vi "overlap_calculator.vi"(0 "T1":dbl min=0.0, 2 "T2":dbl min=0.0, 3 "D":dbl min=0.0) -> (6 "overlap":dbl, 10 "delay":dbl)   [LabVIEW 2015]
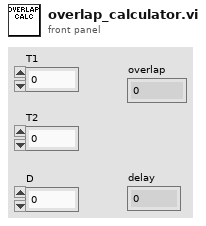
[diagram p1: front panel]
types:
  T1 = enum16{"D<=T1-T2 ^ D<T1", "D<T1 ^ D>T1-T2", "D>=T1"}
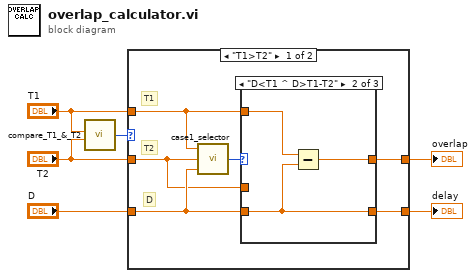
[diagram p0: block diagram]
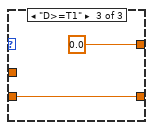
[diagram p3: hidden frame]
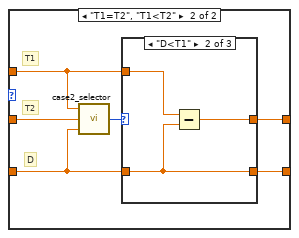
[diagram p4: hidden frame]
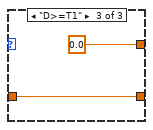
[diagram p6: hidden frame]
diagram:
  n1 = call "compare_T1_&_T2.vi"("T1"="T1", "T2"="T2") -> ("Result"=w2:enum16{"T1>T2", "T1=T2", "T1<T2"})  [unwired: 6 in]
  n2 = case shown="\"T1>T2\"" w2 {
    tunnel: "T1" -> [w10 w23]
    tunnel: "T2" -> [w8 w25]
    tunnel: "D" -> [w9 w21]
    tunnel: [w11 w22] -> w6
    tunnel: [w7 w20] -> w1
    frame "T1>T2" {
      # "D"
      # "T2"
      # "T1"
      n3 = call "case1_selector.vi"("T1"=w10, "T2"=w8, "Delay"=w9) -> ("overlap select"=w12:T1)  [unwired: 4 in]
      n4 = case shown="\"D<T1 ^ D>T1-T2\"" w12 {
        tunnel: w10 -> [_ w17 _]
        tunnel: [w14 w16 0.0] -> w11
        tunnel: w9 -> [w13 w15 w18]
        tunnel: w8 -> [w14 _ _]
        tunnel: [w13 w15 w18] -> w7
        frame "D<=T1-T2 ^ D<T1" {
        }
        frame "D<T1 ^ D>T1-T2" {
          n5 = Subtract(x=w17, y=w15) -> (x-y=w16:dbl)
        }
        frame "D>=T1" {
        }
      }
    }
    frame "T1=T2", "T1<T2" {
      # "D"
      # "T2"
      # "T1"
      n6 = call "case2_selector.vi"("T1"=w23, "T2"=w25, "Delay"=w21) -> ("Case 2 selector"=w24:enum16{"D=0", "D<T1", "D>=T1"})  [unwired: 4 in]
      n7 = case shown="\"D<T1\"" w24 {
        tunnel: w23 -> [w27 w29 _]
        tunnel: [w27 w30 0.0] -> w22
        tunnel: w21 -> [w26 w28 w31]
        tunnel: [w26 w28 w31] -> w20
        frame "D=0" {
        }
        frame "D<T1" {
          n8 = Subtract(x=w29, y=w28) -> (x-y=w30:dbl)
        }
        frame "D>=T1" {
        }
      }
    }
  }
  "overlap" <- w6
  "delay" <- w1
